vi "Tecan Send Command.vi"(7 "Address":u8, 8 "error in (no error)":errorcluster, 10 "Command":string, 11 "VISA resource name in":refnum<visa-resource-name>="COM3") -> (0 "error out":errorcluster, 1 "Status Code":string, 2 "Raw Response":string, 3 "VISA resource name out":refnum<visa-resource-name>, 4 "Value":dbl)   [LabVIEW 2020]
panel:
  out "Timeout":bool
  in  "Timeout(ms)":u32=500
  out "error out 2":errorcluster
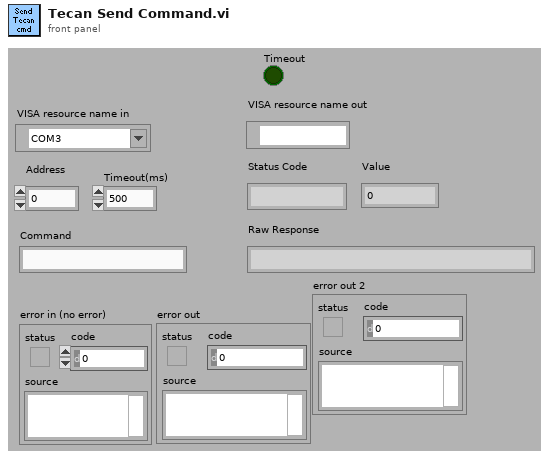
[diagram p1: front panel]
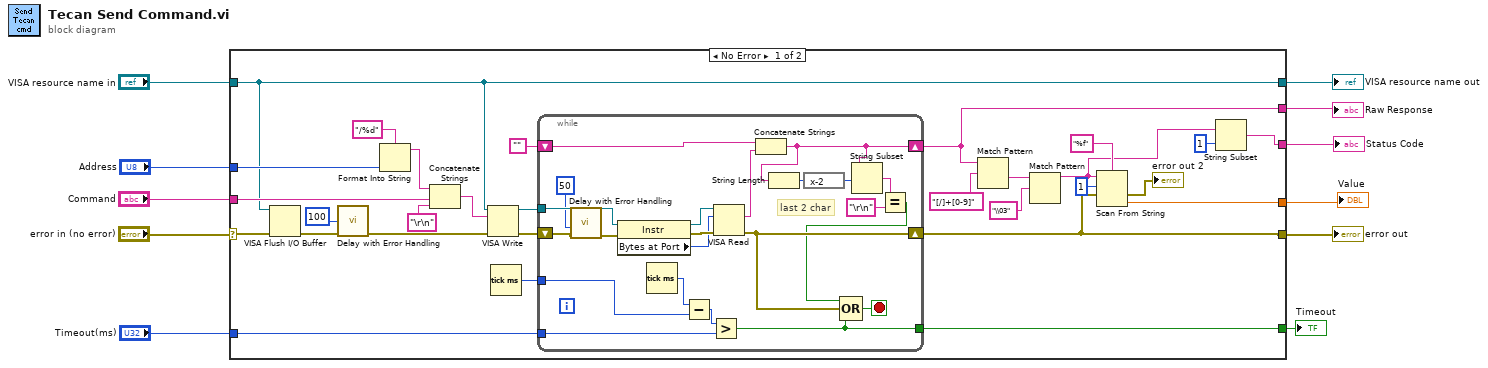
[diagram p0: block diagram]
diagram:
  n1 = case shown="No Error" "error in (no error)" {
    selector: "error in (no error)" -> [w32 w64]
    tunnel: "Command" -> [w36 _]
    tunnel: [w26 w64] -> w9
    tunnel: "VISA resource name in" -> [w16 w63]
    tunnel: [w16 w63] -> w7
    tunnel: [w27 _] -> w6
    tunnel: "Address" -> [w18 _]
    tunnel: [w23 _] -> w5
    tunnel: [w20 _] -> w4
    tunnel: "Timeout(ms)" -> [w15 _]
    tunnel: [w13 _] -> w1
    frame No Error {
      n2 = VISA Flush I/O Buffer(VISA resource name=w16, error in (no error)=w32) -> (error out=w31:errorcluster)  [unwired: 1 in, 1 out]
      n3 = call "Delay with Error Handling.vi"("error in (no error)"=w31, "Delay (ms)"=u32 100) -> ("error out"=w33:errorcluster)  [unwired: 9 in]
      n4 = Format Into String(format string="/%d", w18) -> (resulting string=w35:string)  [unwired: 2 in, 1 out]
      n5 = Concatenate Strings(w35, w36, "\r\n" ("string")) -> (w39:string)
      n6 = VISA Write(VISA resource name=w16, write buffer=w39, error in (no error)=w33) -> (VISA resource name out=w40:refnum<visa-resource-name>, error out=w17:errorcluster)  [unwired: 1 out]
      n7 = Tick Count (ms)() -> (millisecond timer value=w14:u32)
      n8 = while {
        shift-right: [w54] -> w26
        shift-left: w17 -> [w43]
        tunnel: w40 -> [w61]
        tunnel: w15 -> [w55]
        shift-right: [w46] -> w27
        shift-left: "" -> [w51]
        tunnel: [w44] -> w13
        tunnel: w14 -> [w56]
        stop <- w53 stop-if-true
        # "last 2 char"
        n9 = call "Delay with Error Handling.vi"("error in (no error)"=w43, "Delay (ms)"=u32 50 ("milliseconds to wait")) -> ("error out"=w42:errorcluster)  [unwired: 9 in]
        n10 = property class="Instr"(reference=w61, error in=w42) -> (reference out=w60:refnum<visa-resource-name>, error out=w62:errorcluster, "Bytes at Port"=w59:u32)
        n11 = Tick Count (ms)() -> (millisecond timer value=w57:u32)
        n12 = Subtract(x=w57, y=w56) -> (x-y=w58:u32)
        n13 = Greater?(x=w58, y=w55) -> (0:w44:bool)
        n14 = VISA Read(VISA resource name=w60, byte count=w59, error in (no error)=w62) -> (read buffer=w52:string, error out=w54:errorcluster)  [unwired: 2 out]
        n15 = Concatenate Strings(w51, w52) -> (w46:string)
        n16 = String Length(string=w46) -> (length=w47:i32)
        n17 = expression code="x-2"(w47) -> (w45:i32)
        n18 = String Subset(string=w46, offset (0)=w45) -> (substring=w48:string)  [unwired: 1 in]
        n19 = Equal?(x=w48, y="\r\n") -> (x = y?=w49:bool)
        n20 = Compound Arithmetic op=OR(w49, w54, w44) -> (w53:bool)
      }
      n21 = Match Pattern(string=w27, regular expression="[/]+[0-9]") -> (after substring=w29:string)  [unwired: 1 in, 3 out]
      n22 = Match Pattern(string=w29, regular expression="\\03") -> (before substring=w19:string)  [unwired: 1 in, 3 out]
      n23 = Scan From String(format string="%f", input string=w19, initial scan location=u32 1, error in=w26) -> (error out=→"error out 2":errorcluster, output 1=w20:dbl)  [unwired: 1 in, 2 out]
      n24 = String Subset(string=w19, length (rest)=1 ("length (rest)")) -> (substring=w23:string)  [unwired: 1 in]
    }
    frame Error {
    }
  }
  "error out" <- w9
  "Raw Response" <- w6
  "VISA resource name out" <- w7
  "Status Code" <- w5
  "Value" <- w4
  "Timeout" <- w1
